vi "Close EQE.vi"(6 "Skip cell?":bool, 8 "error in (no error)":errorcluster) -> (0 "error out":errorcluster)   [LabVIEW 2011]
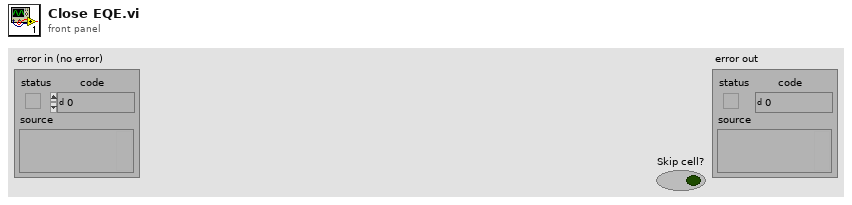
[diagram p1: front panel]
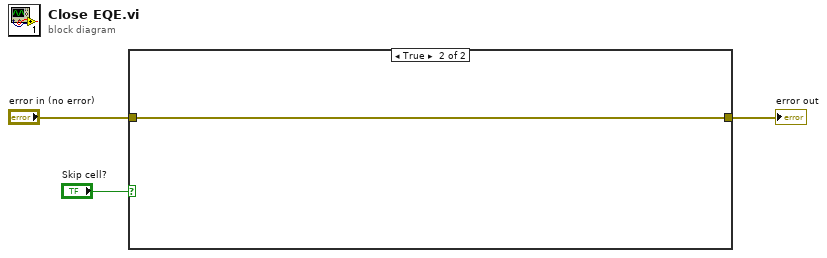
[diagram p0: block diagram]
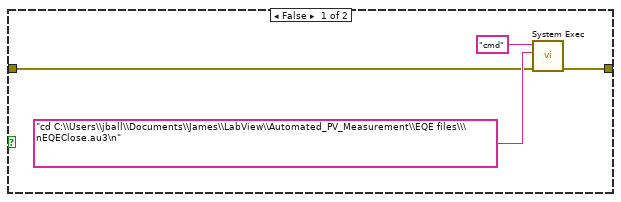
[diagram p2: hidden frame]
diagram:
  n1 = case shown="True" "Skip cell?" {
    tunnel: "error in (no error)" -> [w5 w8]
    tunnel: [w4 w8] -> w1
    frame False {
      n2 = call <vilib>:"System Exec.vi"("error in (no error)"=w5, "standard input"="cd C:\\Users\\jball\\Documents\\James\\LabView\\Automated_PV_Measurement\\EQE files\\\nEQEClose.au3\n", "command line"="cmd") -> ("error out"=w4:errorcluster)  [unwired: 5 in, 3 out]
    }
    frame True {
    }
  }
  "error out" <- w1
